vi "SetTimeOut.vi"(0 "ConnectID":u32, 1 "Timeout (ms)":u32=1000) -> (2 "errorcode":u32, 3 "Err":bool, 4 "Err Msg":string)   [LabVIEW 2011]
uses:
  Windows/System32/Ctccom32v2.dll
panel:
  in  "clear":bool
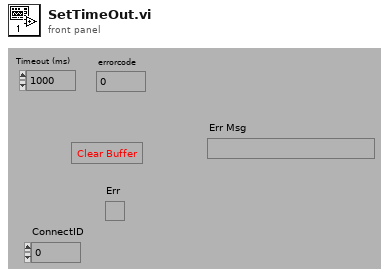
[diagram p1: front panel]
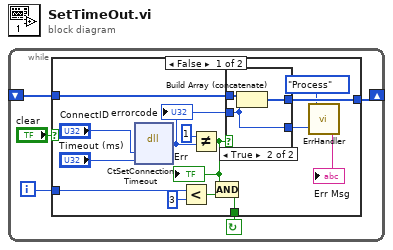
[diagram p0: block diagram]
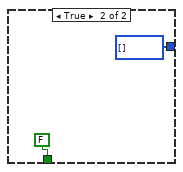
[diagram p3: hidden frame]
diagram:
  n1 = while {
    shift-left: _ -> [w3]
    shift-right: [w2] -> _
    i -> [w4]
    stop <- w5 continue-if-true
    n2 = case shown="False" "clear" {
      tunnel: [w16 FALSE] -> w5
      tunnel: w4 -> [w9 _]
      tunnel: w3 -> [w15 _]
      tunnel: [w14 u16[] []] -> w2
      frame False {
        n3 = dll-call lib="C:/WINNT/system32/CtcEmcorev2.dll" fn="CtSetConnectionTimeout" label="CtGetRegister"("ConnectID"="ConnectID", "MSecond"="Timeout (ms)") -> (w17:u32)  [unwired: 5 in, 2 out]
        "errorcode" <- w17
        n4 = Less?(x=w9, y=3) -> (x < y?=w7:bool)
        n5 = Not Equal?(x=u16 1, y=w17) -> (x != y?=w13:bool)
        "Err" <- w13
        n6 = Compound Arithmetic op=AND(w13, w7) -> (w16:bool)
        n7 = case shown="True" w13 {
          tunnel: w17 -> [w20 w22]
          tunnel: [w21 w23] -> w14
          tunnel: w15 -> [w21 w24]
          tunnel: [w20 w22] -> w11
          frame False {
          }
          frame True {
            n8 = Build Array (concatenate)(w24, w22) -> (w23:u32[])
          }
        }
        n9 = call "ErrHandler.vi"("Err Code"=w11, "Action"=enum16{"Init", "Process"}."Process") -> ("Err Msg"=→"Err Msg":string)
      }
      frame True {
      }
    }
  }
